vi "test_connection_faildialog.vi"(8 "error in (no error)":errorcluster caption="エラー入力（エラーなし）", 9 "想定レスポンス":string="LC\r", 10 "コマンド":string="YSSL\n\r", 11 "VISAリソース名":refnum<visa-resource-name>) -> (0 "error out":errorcluster caption="エラー出力", 2 "connected?":bool)   [LabVIEW 2017]
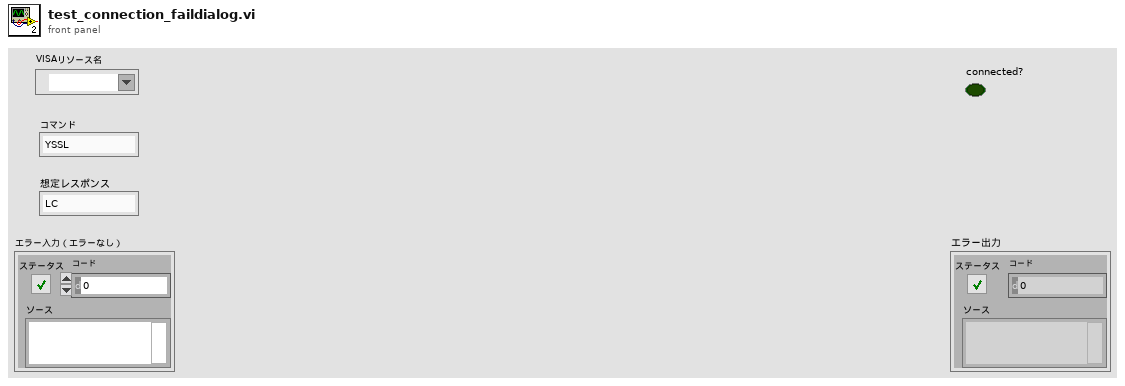
[diagram p1: front panel]
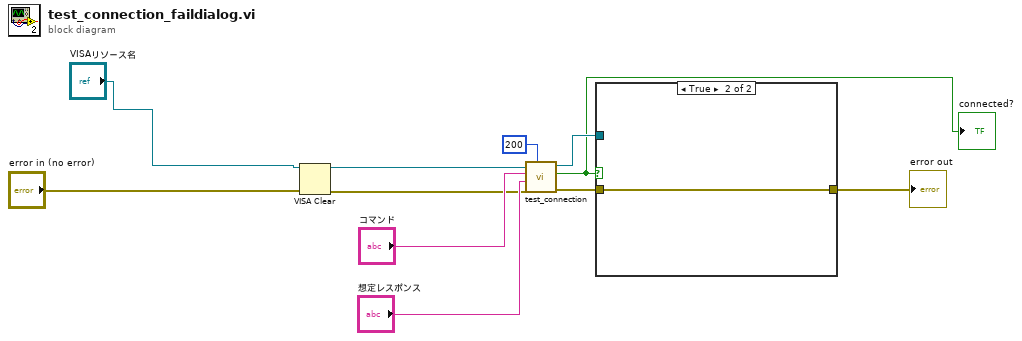
[diagram p0: block diagram]
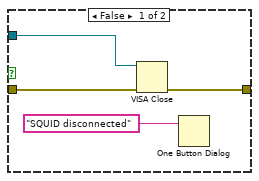
[diagram p2: hidden frame]
diagram:
  n1 = VISA Clear(VISA resource name="VISAリソース名", error in (no error)="error in (no error)") -> (VISA resource name out=w7:refnum<visa-resource-name>, error out=w6:errorcluster)
  n2 = call "test_connection.vi"("文字送信間隔 (500 ms)"=200, "error in (no error)"=w6, "想定レスポンス"="想定レスポンス", "コマンド"="コマンド", "VISAリソース名"=w7) -> ("error out"=w9:errorcluster, "一致？"=w3:bool, "VISAリソース名 （出力）"=w8:refnum<visa-resource-name>)  [unwired: 3 in, 1 out]
  "connected?" <- w3
  n3 = case shown="TRUE" w3 {
    tunnel: w9 -> [w15 w16]
    tunnel: w8 -> [w14 _]
    tunnel: [w12 w16] -> w4
    frame False {
      n4 = VISA Close(VISA resource name=w14, error in (no error)=w15) -> (error out=w12:errorcluster)
      n5 = One Button Dialog(message="SQUID disconnected") -> ()  [unwired: 1 in, 1 out]
    }
    frame True {
    }
  }
  "error out" <- w4
